vi "To Speed.vi"(2 "error in (no error)":errorcluster, 3 "Motor PWM":dbl, 4 "Car.lvclass":refnum<class "Car.lvclass">) -> (0 "error out":errorcluster, 1 "Speed":dbl)   [LabVIEW 2015, in "Car.lvclass"]
uses:
  Car.lvclass
  Car.lvclass/Car.ctl
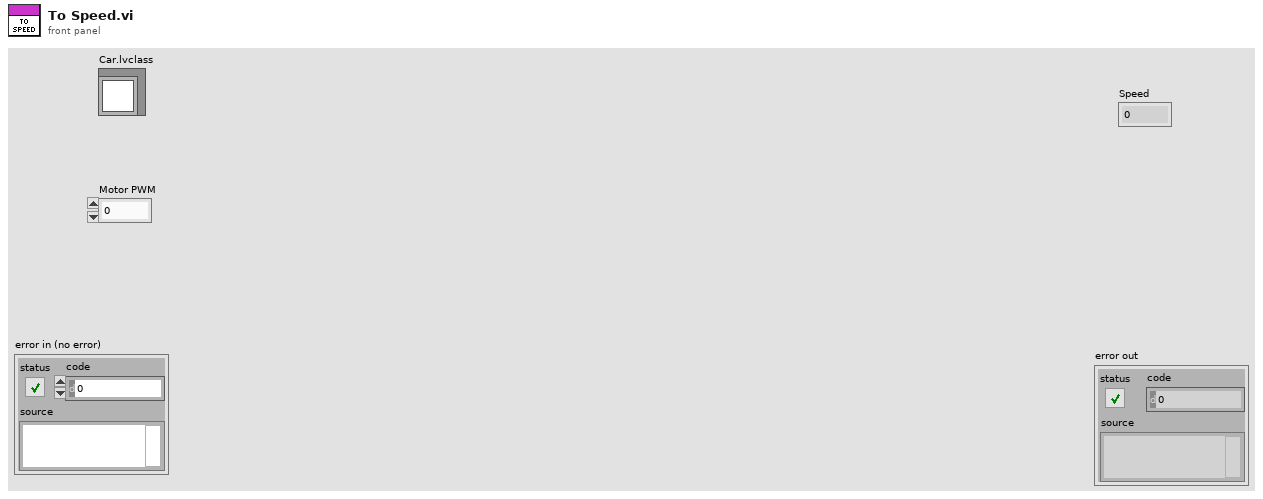
[diagram p1: front panel]
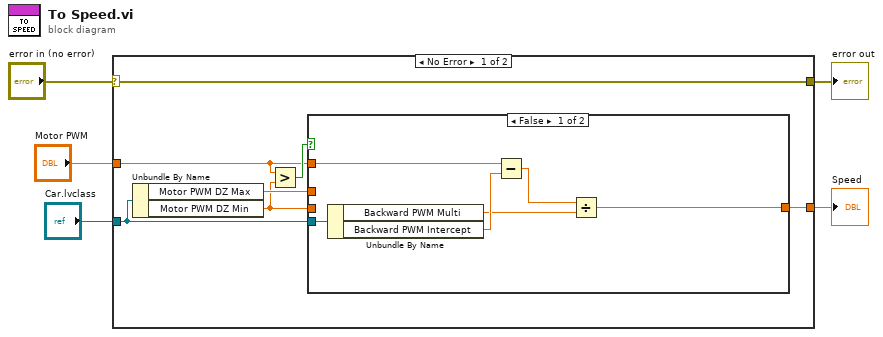
[diagram p0: block diagram]
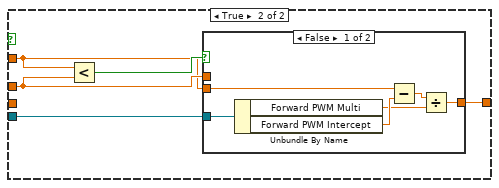
[diagram p2: hidden frame]
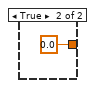
[diagram p3: hidden frame]
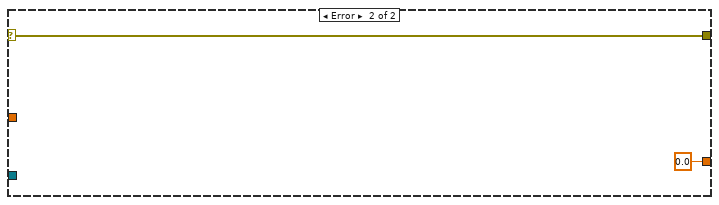
[diagram p4: hidden frame]
diagram:
  n1 = case shown="No Error" "error in (no error)" {
    selector: "error in (no error)" -> [w12 w32]
    tunnel: [w12 w32] -> w4
    tunnel: [w8 0.0] -> w3
    tunnel: "Car.lvclass" -> [w7 _]
    tunnel: "Motor PWM" -> [w9 _]
    frame No Error {
      n2 = Unbundle By Name(w7) -> ("Motor PWM DZ Max"=w10:dbl, "Motor PWM DZ Min"=w6:dbl)
      n3 = Greater?(x=w9, y=w6) -> (0:w11:bool)
      n4 = case shown="False" w11 {
        tunnel: w10 -> [_ w20]
        tunnel: w9 -> [w16 w19]
        tunnel: [w13 w22] -> w8
        tunnel: w7 -> [w18 w21]
        tunnel: w6 -> [_ _]
        frame False {
          n5 = Unbundle By Name(w18) -> ("Backward PWM Multi"=w15:dbl, "Backward PWM Intercept"=w17:dbl)
          n6 = Subtract(x=w16, y=w17) -> (x-y=w14:dbl)
          n7 = Divide(x=w14, y=w15) -> (x/y=w13:dbl)
        }
        frame True {
          n8 = Less?(x=w19, y=w20) -> (x < y?=w23:bool)
          n9 = case shown="False" w23 {
            tunnel: [w24 0.0] -> w22
            tunnel: w21 -> [w29 _]
            tunnel: w20 -> [_ _]
            tunnel: w19 -> [w27 _]
            frame False {
              n10 = Unbundle By Name(w29) -> ("Forward PWM Multi"=w25:dbl, "Forward PWM Intercept"=w28:dbl)
              n11 = Subtract(x=w27, y=w28) -> (x-y=w26:dbl)
              n12 = Divide(x=w26, y=w25) -> (x/y=w24:dbl)
            }
            frame True {
            }
          }
        }
      }
    }
    frame Error {
    }
  }
  "Speed" <- w3
  "error out" <- w4
